vi "communicateVSSRefPlacement.vi"(6 "SEND?":bool, 8 "error in (no error)":errorcluster, 9 "VSSRef Replacement infos":T1={"Local IP:"="192.168.0.102", "Port"=10003, "Server IP:"="224.5.23.2"}, 10 "Game":refnum<class "Game.lvclass">, 11 "Communication in":refnum<class "Communication.lvclass">) -> (0 "error out":errorcluster, 3 "Communication out":refnum<class "Communication.lvclass">)   [LabVIEW 2023, in "Communication.lvclass"]
uses:
  Communication.lvclass
  Game_class/Game.lvclass
  Controls/vision_control.ctl
  Game_class/Game.lvclass/Game.ctl
  Game_class/Read KeeperTeam.vi
  Game_class/Read AllyRef.vi
  Ally_class/Ally.lvclass
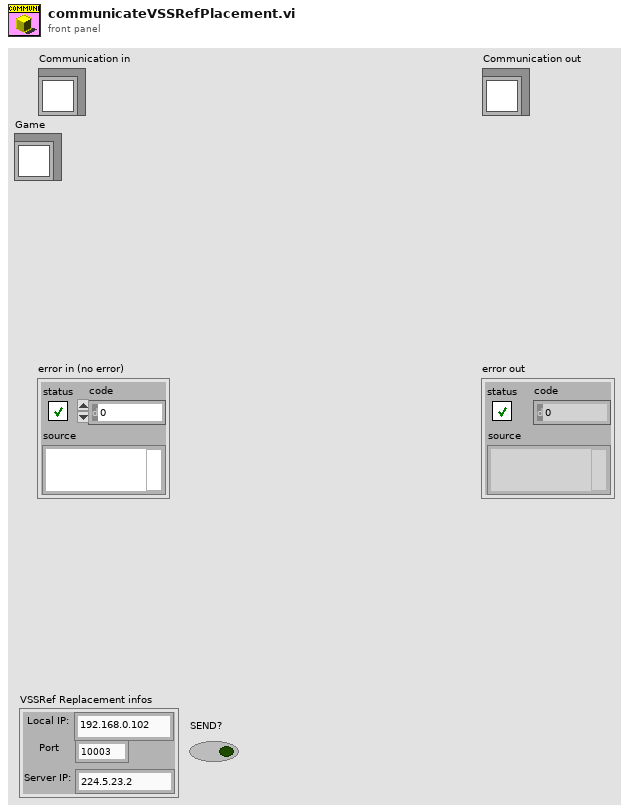
[diagram p1: front panel]
types:
  T1 = typedef "vision_control.ctl" = cluster{"Local IP:":string, "Port":i32, "Server IP:":string}
  T2 = cluster{"id":i32, "x":dbl, "y":dbl, "orientation":dbl}[]
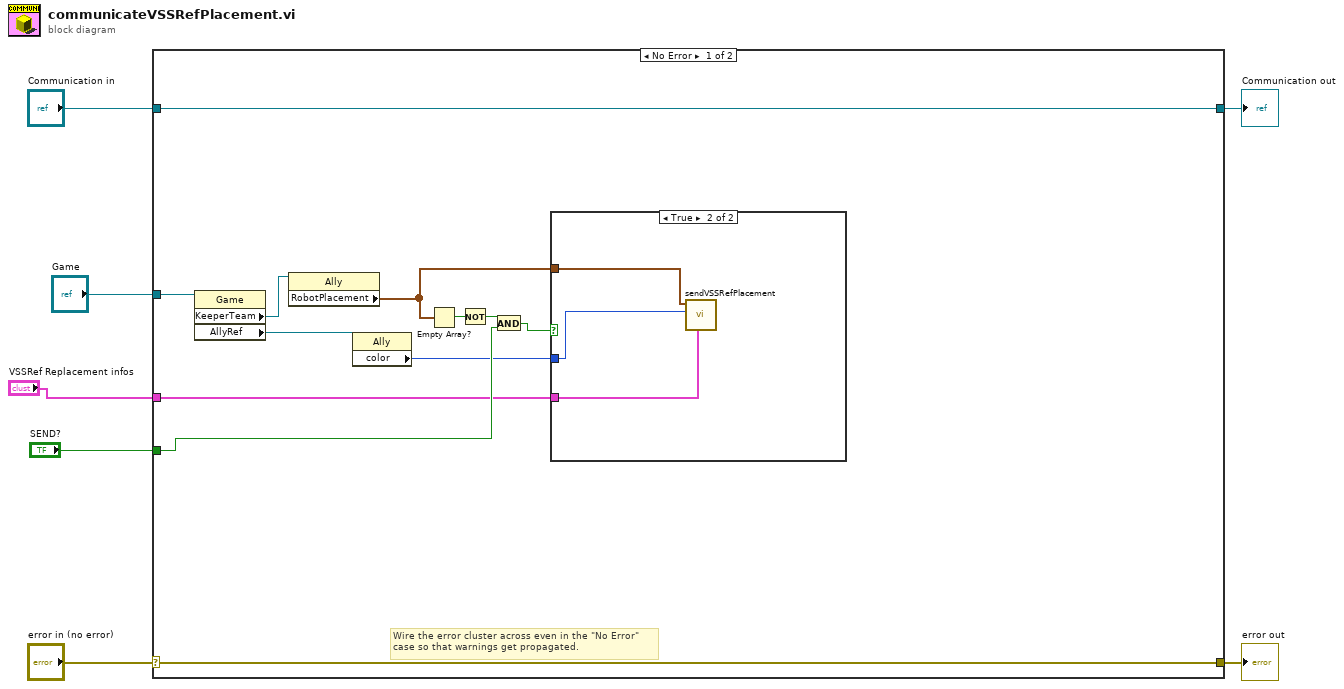
[diagram p0: block diagram]
diagram:
  n1 = case shown="No Error" "error in (no error)" {
    selector: "error in (no error)" -> [w18 w24]
    tunnel: [w18 w24] -> w6
    tunnel: [w19 w23] -> w4
    tunnel: "Communication in" -> [w19 w23]
    tunnel: "Game" -> [w17 _]
    tunnel: "VSSRef Replacement infos" -> [w12 _]
    tunnel: "SEND?" -> [w14 _]
    frame No Error {
      # "Wire the error cluster across even in the \"No Error\"\ncase so that warnings get propagated."
      n2 = property class="Game"(reference=w17) -> ("KeeperTeam"=w9:refnum<class "Ally.lvclass">, "AllyRef"=w11:refnum<class "Ally.lvclass">)  [unwired: 1 in, 2 out]
      n3 = property class="Ally"(reference=w9) -> ("RobotPlacement"=w8:T2)  [unwired: 1 in, 2 out]
      n4 = property class="Ally"(reference=w11) -> ("color"=w10:enum16{"Azul", "Amarelo"})  [unwired: 1 in, 2 out]
      n5 = Empty Array?(array=w8) -> (empty?=w16:bool)
      n6 = Not(x=w16) -> (.not. x?=w15:bool)
      n7 = And(x=w15, y=w14) -> (x .and. y?=w13:bool)
      n8 = case shown="True" w13 {
        tunnel: w8 -> [_ w22]
        tunnel: w12 -> [_ w20]
        tunnel: w10 -> [_ w21]
        frame False {
        }
        frame True {
          n9 = call "sendVSSRefPlacement.vi"("VSSRef Replacement infos"=w20, "color"=w21, "RobotPlacement"=w22) -> ()  [unwired: 8 in]
        }
      }
    }
    frame Error {
    }
  }
  "error out" <- w6
  "Communication out" <- w4
